vi "Theta 0.vi"(7 "XYZ_6":dbl[](array[numeric])=[0.0, 0.0, 0.0], 11 "6R Type 3 Serial Arm Class.lvclass":refnum<class "NI_Robotics_6R Type 3 Serial Arm Class.lvclass">) -> (1 "valid?":bool, 2 "theta_0 array":dbl[](array[numeric]), 3 "6R Type 3 Serial Arm Class.lvclass out":refnum<class "NI_Robotics_6R Type 3 Serial Arm Class.lvclass">)   [LabVIEW 2017, in "NI_Robotics_6R Type 3 Serial Arm Class.lvclass"]
uses:
  <vilib>/robotics/Kinematics/Analytical/6R/Type 3/NI_Robotics_6R Type 3 Serial Arm Class.lvclass
  c:/Program Files (x86)/National Instruments/LabVIEW 2017/vi.lib/robotics/Kinematics/Analytical/Generic/NI_Robotics_Analytical Serial Arm Class.lvclass
  <vilib>/robotics/Kinematics/Link/NI_Robotics_Link.lvclass/NI_Robotics_Link.ctl
  <vilib>/robotics/Kinematics/Link/Get Kinematic Parameters.vi
  <vilib>/robotics/Kinematics/Analytical/Generic/NI_Robotics_Analytical Serial Arm Class.lvclass
  c:/Program Files (x86)/National Instruments/LabVIEW 2017/vi.lib/robotics/Kinematics/Robot/NI_Robotics_Serial Robot Arm.lvclass
  <vilib>/robotics/Kinematics/Analytical/Generic/Accessors/Read alpha_n0.vi
  <vilib>/robotics/Kinematics/Robot/Get Links.vi
  <vilib>/robotics/Kinematics/Analytical/NI_Robotics_AnalyticKinematics.lvlib
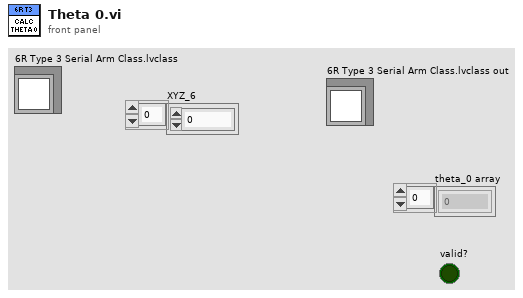
[diagram p1: front panel]
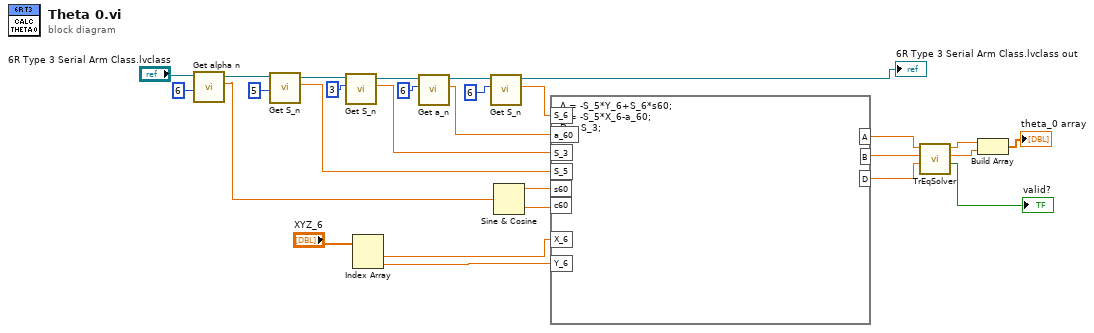
[diagram p0: block diagram]
diagram:
  n1 = call <vilib>:"Get alpha n.vi"("n"=6, "Analytical Serial Arm Class in"="6R Type 3 Serial Arm Class.lvclass") -> ("alpha n"=w18:dbl, "Analytical Serial Arm Class out"=w26:refnum<class "NI_Robotics_6R Type 3 Serial Arm Class.lvclass">)  [unwired: 8 in]
  n2 = call <vilib>:"Get S_n.vi"("n"=5, "Analytical Serial Arm Class in"=w26) -> ("S_n"=w17:dbl, "Analytical Serial Arm Class out"=w24:refnum<class "NI_Robotics_6R Type 3 Serial Arm Class.lvclass">)  [unwired: 8 in]
  n3 = call <vilib>:"Get S_n.vi"("n"=3, "Analytical Serial Arm Class in"=w24) -> ("S_n"=w16:dbl, "Analytical Serial Arm Class out"=w22:refnum<class "NI_Robotics_6R Type 3 Serial Arm Class.lvclass">)  [unwired: 8 in]
  n4 = Index Array(array="XYZ_6") -> (element #1=w13:dbl, element #2=w12:dbl)  [unwired: 2 in]
  n5 = call <vilib>:"Get a_n.vi"("n"=6, "Analytical Serial Arm Class in"=w22) -> ("a_n"=w15:dbl, "Analytical Serial Arm Class out"=w4:refnum<class "NI_Robotics_6R Type 3 Serial Arm Class.lvclass">)  [unwired: 8 in]
  n6 = call <vilib>:"Get S_n.vi"("n"=6, "Analytical Serial Arm Class in"=w4) -> ("S_n"=w1:dbl, "Analytical Serial Arm Class out"=→"6R Type 3 Serial Arm Class.lvclass out":refnum<class "NI_Robotics_6R Type 3 Serial Arm Class.lvclass">)  [unwired: 8 in]
  n7 = Sine & Cosine(0:w18) -> (1:w20:dbl, 2:w19:dbl)
  n8 = formula code="A = -S_5*Y_6+S_6*s60;\nB = -S_5*X_6-a_60;\nD = S_3;"("a_60"=w15, "S_3"=w16, "S_5"=w17, "s60"=w20, "c60"=w19, "X_6"=w13, "Y_6"=w12, "S_6"=w1) -> ("A"=w11:dbl, "B"=w10:dbl, "D"=w9:dbl)
  n9 = call <vilib>:"TrEqSolver.vi"("D"=w9, "B"=w10, "A"=w11) -> ("Solution Exists"=→"valid?":bool, "angle 2"=w6:dbl, "angle 1"=w7:dbl)  [unwired: 6 in]
  n10 = Build Array(w7, w6) -> (→"theta_0 array":dbl[])
